vi "MSEncoder Case-5-UpdConj.vi"(8 "error in (no error)":errorcluster, 9 "ParamValIn":variant, 11 "MSEncoder in":refnum<class "MSEncoder.lvclass">) -> (0 "error out":errorcluster, 3 "MSEncoder out":refnum<class "MSEncoder.lvclass">)   [LabVIEW 2018, in "MSEncoder.lvclass"]
uses:
  MSEncoder.lvclass
  Ctl/MSEditorParam updConj.ctl
  MSEncoder.lvclass/MSEncoder.ctl
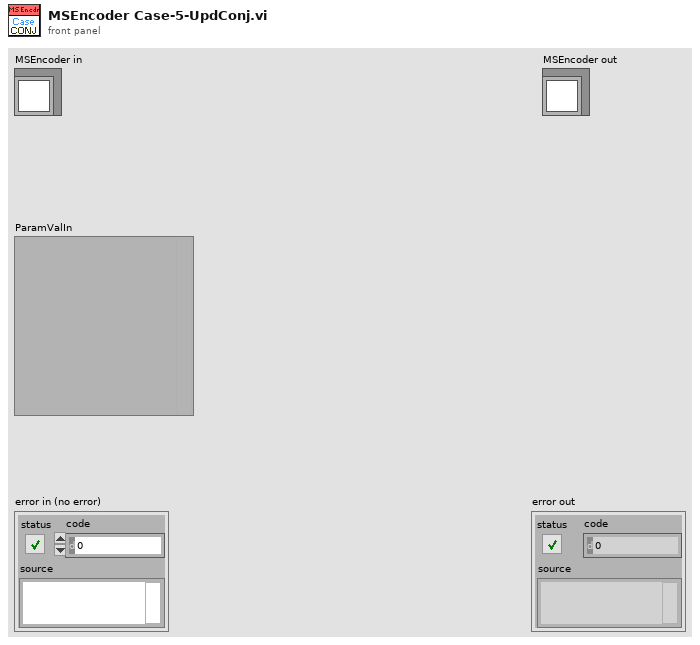
[diagram p1: front panel]
types:
  T1 = typedef "MSEditorParam updConj.ctl" = cluster{"iniPhase":u32, "conjLen":ext[], "phaseDiff":u64[], "fixedLen":bool}
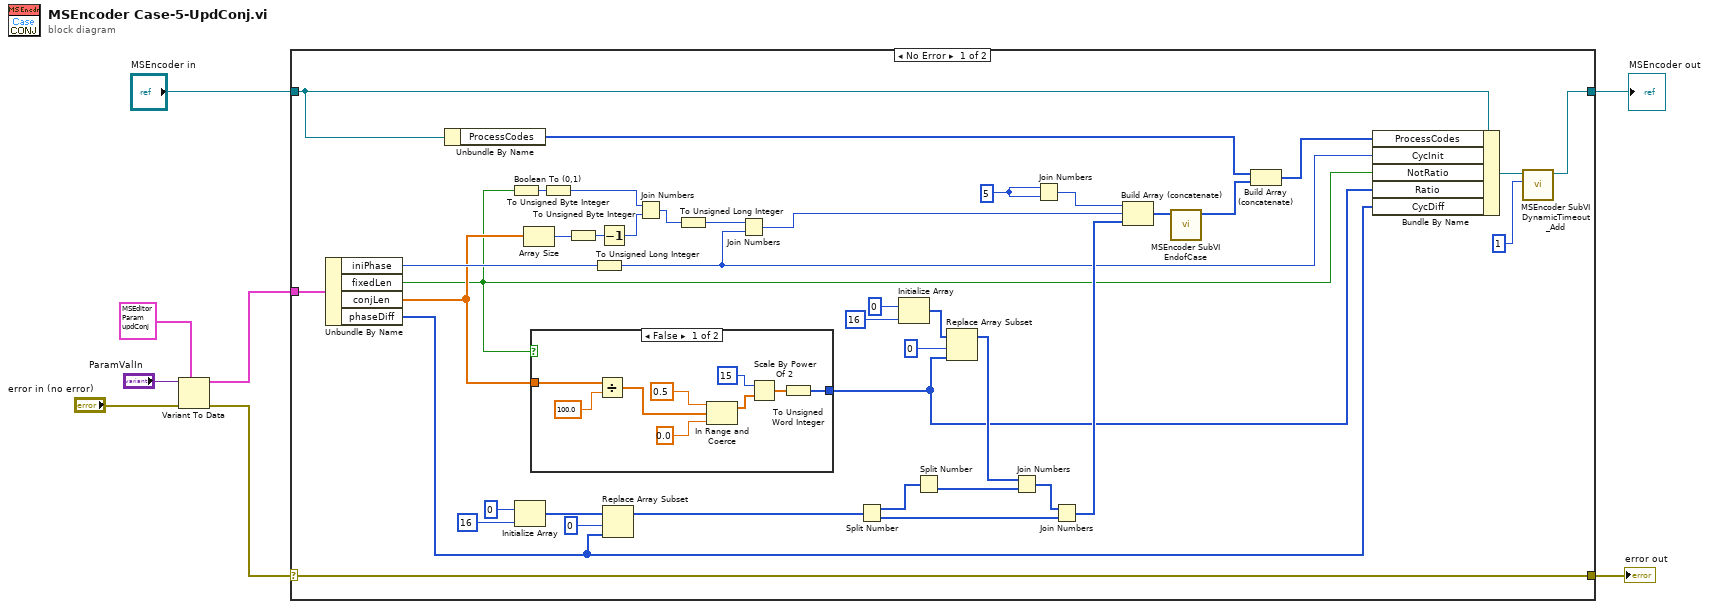
[diagram p0: block diagram]
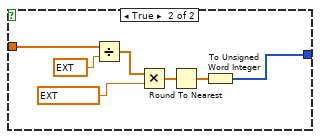
[diagram p2: hidden frame]
diagram:
  n1 = Variant To Data(error in="error in (no error)", type=T1 {"iniPhase"=2147483648, "conjLen"=[3.0, 3.0], "phaseDiff"=[2147483648, 2147483648], "fixedLen"=FALSE} ("ParamValueType"), Variant="ParamValIn") -> (data=w2:T1, error out=w1:errorcluster)
  n2 = case shown="No Error" w1 {
    selector: w1 -> [w48 w67]
    tunnel: "MSEncoder in" -> [w49 w66]
    tunnel: [w48 w67] -> w8
    tunnel: [w9 w66] -> w6
    tunnel: w2 -> [w24 _]
    frame No Error {
      w47 = u32 5
      n3 = Unbundle By Name(w24) -> ("iniPhase"=w26:u32, "fixedLen"=w17:bool, "conjLen"=w20:ext[], "phaseDiff"=w25:u64[])
      n4 = Unbundle By Name(w49) -> ("ProcessCodes"=w23:u64[])
      n5 = Boolean To (0,1)(Boolean=w17) -> (0, 1=w16:i16)
      n6 = Initialize Array(u64 0, 16 ("dimension size")) -> (w34:u64[])
      n7 = Array Size(array=w20) -> (size(s)=w41:i32)
      n8 = case shown="False" w17 {
        tunnel: w20 -> [w51 w65]
        tunnel: [w50 w59] -> w18
        frame False {
          n9 = Divide(x=w51, y=100.0) -> (x/y=w58:ext[])
          n10 = In Range and Coerce(upper limit=0.5, x=w58, lower limit=0.0) -> (coerced(x)=w55:ext[])  [unwired: 1 out]
          n11 = Scale By Power Of 2(n=i16 15, x=w55) -> (x*2^n=w53:ext[])
          n12 = To Unsigned Word Integer(number=w53) -> (unsigned 16bit integer=w50:u16[])
        }
        frame True {
          n13 = Divide(x=w65, y=ext 1000.0) -> (x/y=w62:ext[])
          n14 = Multiply(x=w62, y=ext 40000000.0) -> (x*y=w61:ext[])
          n15 = Round To Nearest(number=w61) -> (nearest integer value=w60:ext[])
          n16 = To Unsigned Word Integer(number=w60) -> (unsigned 16bit integer=w59:u16[])
        }
      }
      n17 = To Unsigned Byte Integer(number=w16) -> (unsigned 8bit integer=w14:u8)
      n18 = To Unsigned Byte Integer(number=w41) -> (unsigned 8bit integer=w27:u8)
      n19 = To Unsigned Long Integer(number=w26) -> (unsigned 32bit integer=w37:u32)
      n20 = Decrement(x=w27) -> (x-1=w15:u8)
      n21 = Replace Array Subset(array=w34, new element=w25, index=0) -> (w32:u64[])
      n22 = Join Numbers(hi=w14, lo=w15) -> ((hi.lo)=w13:u16)
      n23 = To Unsigned Long Integer(number=w13) -> (unsigned 32bit integer=w12:u32)
      n24 = Join Numbers(hi=w12, lo=w37) -> ((hi.lo)=w40:u64)
      n25 = Split Number(x=w32) -> (hi(x)=w45:u32[], lo(x)=w42:u32[])
      n26 = Initialize Array(u16 0, 16 ("dimension size")) -> (w31:u16[])
      n27 = Split Number(x=w45) -> (lo(x)=w44:u16[])  [unwired: 1 out]
      n28 = Replace Array Subset(array=w31, new element=w18, index=0) -> (w19:u16[])
      n29 = Join Numbers(hi=w19, lo=w44) -> ((hi.lo)=w43:u32[])
      n30 = Join Numbers(hi=w47, lo=w47) -> ((hi.lo)=w46:u64)
      n31 = Join Numbers(hi=w43, lo=w42) -> ((hi.lo)=w39:u64[])
      n32 = Build Array (concatenate)(w46, w40, w39) -> (w38:u64[])
      n33 = call "MSEncoder SubVI EndofCase.vi"("Case codes"=w38) -> ("Case codes with end"=w21:u64[])  [unwired: 9 in, 1 out]
      n34 = Build Array (concatenate)(w23, w21) -> (w22:u64[])
      n35 = Bundle By Name(cluster=w49, "ProcessCodes"=w22, "CycInit"=w37, "NotRatio"=w17, "Ratio"=w18, "CycDiff"=w25) -> (w11:refnum<class "MSEncoder.lvclass">)
      n36 = call "MSEncoder SubVI DynamicTimeout_Add.vi"("Timeout_ms"=1, "MSEncoder"=w11) -> ("MSEncoder"=w9:refnum<class "MSEncoder.lvclass">)  [unwired: 8 in, 1 out]
    }
    frame Error {
    }
  }
  "error out" <- w8
  "MSEncoder out" <- w6
